vi "MicroPVHTML100_1.vi"(10 "path in":path, 11 "network":path) -> (2 "Chemin du fichier":path, 3 "Chemin du fichier 2":path)   [LabVIEW 2020]
panel:
  out "sortie d'erreur":errorcluster
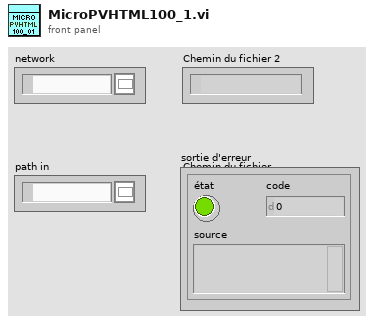
[diagram p1: front panel]
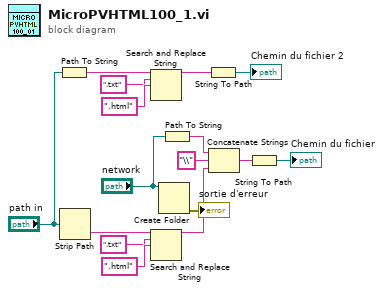
[diagram p0: block diagram]
diagram:
  n1 = Path To String(path="path in") -> (string=w2:string)
  n2 = Strip Path(path="path in") -> (name=w11:string)  [unwired: 1 out]
  n3 = Search and Replace String(input string=w2, search string=".txt" ("chaîne recherchée"), replace string=".html" ("chaîne de remplacement (\"\")")) -> (result string=w5:string)  [unwired: 5 in, 3 out]
  n4 = Search and Replace String(input string=w11, search string=".txt" ("chaîne recherchée"), replace string=".html" ("chaîne de remplacement (\"\")")) -> (result string=w14:string)  [unwired: 5 in, 3 out]
  n5 = Create Folder ("Créer un dossier")(path (use dialog)="network") -> (error out=→"sortie d'erreur":errorcluster)  [unwired: 2 in, 2 out]
  n6 = Path To String(path="network") -> (string=w12:string)
  n7 = String To Path(string=w5) -> (path=→"Chemin du fichier 2":path)
  n8 = Concatenate Strings(w12, "\\" ("chaîne"), w14) -> (w15:string)
  n9 = String To Path(string=w15) -> (path=→"Chemin du fichier":path)
